vi "Configure.vi"(11 "Neopixel - FPGA In":refnum<class "Neopixel - FPGA.lvclass">) -> (2 "Timed Out?":bool, 3 "Neopixel - FPGA Out":refnum<class "Neopixel - FPGA.lvclass">)   [LabVIEW 2021, in "Neopixel - FPGA.lvclass"]
uses:
  Neopixel - FPGA.lvclass
  Neopixel - FPGA.lvclass/Neopixel - FPGA.ctl
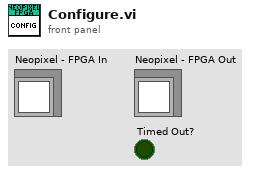
[diagram p1: front panel]
types:
  T1 = typedef "Neopixel Shared.lvlib/Neopixel FIFO Command.ctl" = enum8{"Set Number Of Neopixels", "Update Frame"}
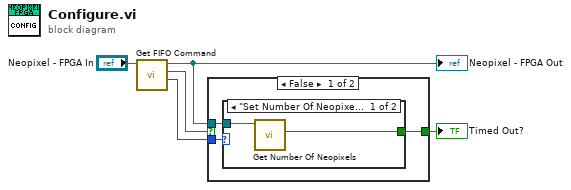
[diagram p0: block diagram]
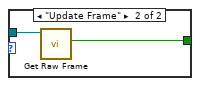
[diagram p2: hidden frame]
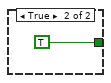
[diagram p3: hidden frame]
diagram:
  n1 = call "Get FIFO Command.vi"("Neopixel - FPGA In"="Neopixel - FPGA In") -> ("Command"=w2:T1, "Timed Out?"=w3:bool, "Neopixel - FPGA Out"=w1:refnum<class "Neopixel - FPGA.lvclass">)  [unwired: 8 in]
  "Neopixel - FPGA Out" <- w1
  n2 = case shown="False" w3 {
    tunnel: w2 -> [w8 _]
    tunnel: [w7 TRUE ("Timed Out?")] -> w5
    tunnel: w1 -> [w6 _]
    frame False {
      n3 = case shown="\"Set Number Of Neopixels\"" w8 {
        tunnel: [w10 w12] -> w7
        tunnel: w6 -> [w9 w11]
        frame "Set Number Of Neopixels" {
          n4 = call "Get Number Of Neopixels.vi"("Neopixel - FPGA In"=w9) -> ("Timed Out?"=w10:bool)  [unwired: 9 in, 1 out]
        }
        frame "Update Frame" {
          n5 = call "Get Raw Frame.vi"("Neopixel - FPGA In"=w11) -> ("Timed Out?"=w12:bool)  [unwired: 9 in, 1 out]
        }
      }
    }
    frame True {
    }
  }
  "Timed Out?" <- w5
